vi "Test read SPI.vi"() -> ()   [LabVIEW 2012]
uses:
  <vilib>/ni845x/ni845x.llb/ni845xControl.ctl
panel:
  out "dt":u32
  out "Waveform Chart":T1(graph)
  in  "accel range (g)":u16(ring)=2 caption="Accelerometer range (g)" items=["2"=2, "4"=4, "8"=8, "16"=16]
  in  "gyro range (deg/sec)":u16(ring)=250 caption="Gyro range (deg/sec)" items=["250"=250, "500"=500, "1000"=1000, "2000"=2000]
  in  "Stop":bool
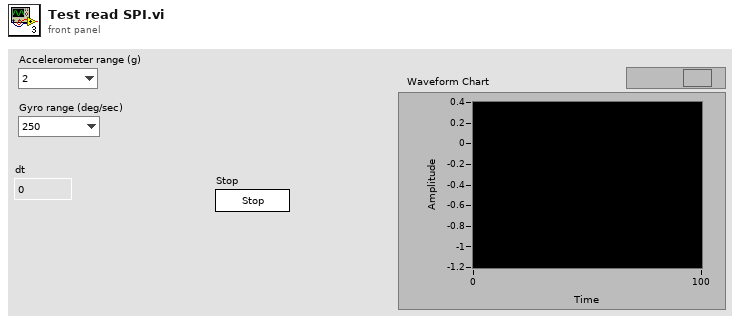
[diagram p1: front panel]
types:
  T1 = cluster{"Accel[0]":dbl, "Accel[1]":dbl, "Accel[2]":dbl, "Accel[3]":dbl, "Accel[4]":dbl, "Accel[5]":dbl, "Accel[6]":dbl, "Accel[7]":dbl, "Accel[8]":dbl}
  T2 = typedef "ni845xControl.ctl" = refnum<k21>
  T3 = typedef "AccelerometerSPI.ctl" = cluster{"Device":T2, "spi configuration":T4}
  T4 = typedef "ni845xSpiConfiguration.ctl" = refnum<k20>
  T5 = typedef "Accelerometer Data.ctl" = cluster{"Accel":dbl[], "Gyro":dbl[], "Time":u64, "Trigger":bool}
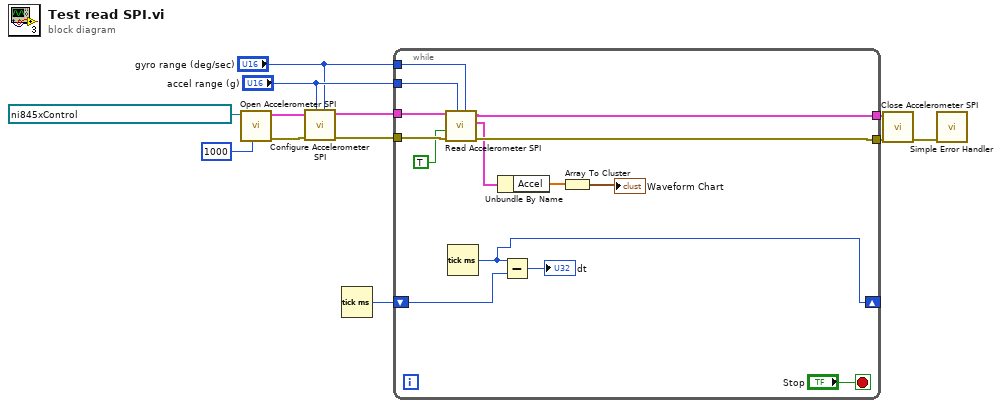
[diagram p0: block diagram]
diagram:
  n1 = call "Open Accelerometer SPI.vi"("Clock Rate in kHz"=u16 1000, "Device"=T2 "USB0::0x3923::0x7166::01879089::RAW") -> ("error out"=w6:errorcluster, "Accelerometer"=w7:T3)  [unwired: 8 in]
  n2 = call "Configure Accelerometer SPI.vi"("gyro range (deg/sec)"="gyro range (deg/sec)", "accel range (g)"="accel range (g)", "error in (no error)"=w6, "Accelerometer"=w7) -> ("error out"=w4:errorcluster, "Accelerometer out"=w5:T3)  [unwired: 6 in]
  n3 = Tick Count (ms)() -> (millisecond timer value=w1:u32)
  n4 = while {
    tunnel: [w20] -> w9
    tunnel: [w19] -> w8
    tunnel: w5 -> [w25]
    tunnel: w4 -> [w24]
    tunnel: "accel range (g)" -> [w23]
    tunnel: "gyro range (deg/sec)" -> [w22]
    shift-right: [w14] -> _
    shift-left: w1 -> [w15]
    stop <- "Stop" stop-if-true
    n5 = call "Read Accelerometer SPI.vi"("gyro range (deg/sec)"=w22, "accel range (g)"=w23, "error in (no error)"=w24, "check ready"=TRUE, "Accelerometer"=w25) -> ("error out"=w19:errorcluster, "Accelerometer Data"=w18:T5, "Accelerometer out"=w20:T3)  [unwired: 3 in, 1 out]
    n6 = Tick Count (ms)() -> (millisecond timer value=w14:u32)
    n7 = Unbundle By Name(w18) -> ("Accel"=w17:dbl[])
    n8 = Subtract(x=w14, y=w15) -> (x-y=→"dt":u32)
    n9 = Array To Cluster(array=w17) -> (cluster=→"Waveform Chart":T1)
  }
  n10 = call "Close Accelerometer SPI.vi"("error in (no error)"=w8, "Accelerometer"=w9) -> ("error out"=w10:errorcluster)  [unwired: 9 in]
  n11 = call <vilib>:"Simple Error Handler.vi"("error in (no error)"=w10) -> ()  [unwired: 4 in, 5 out]
